vi "winHost.vi"() -> ()   [LabVIEW 2017]
uses:
  <vilib>/Utility/file.llb/Write Delimited Spreadsheet (DBL).vi
panel:
  in  "file path (dialog if empty)":path=path "C:/Users/adamg/Desktop/testdata137deg.csv"
  in  "Orientation":dbl
  in  "Force":dbl
  in  "Save":bool
  in  "stop":bool
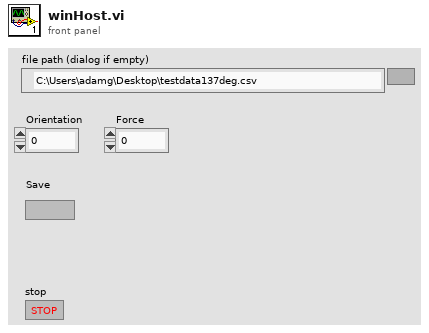
[diagram p1: front panel]
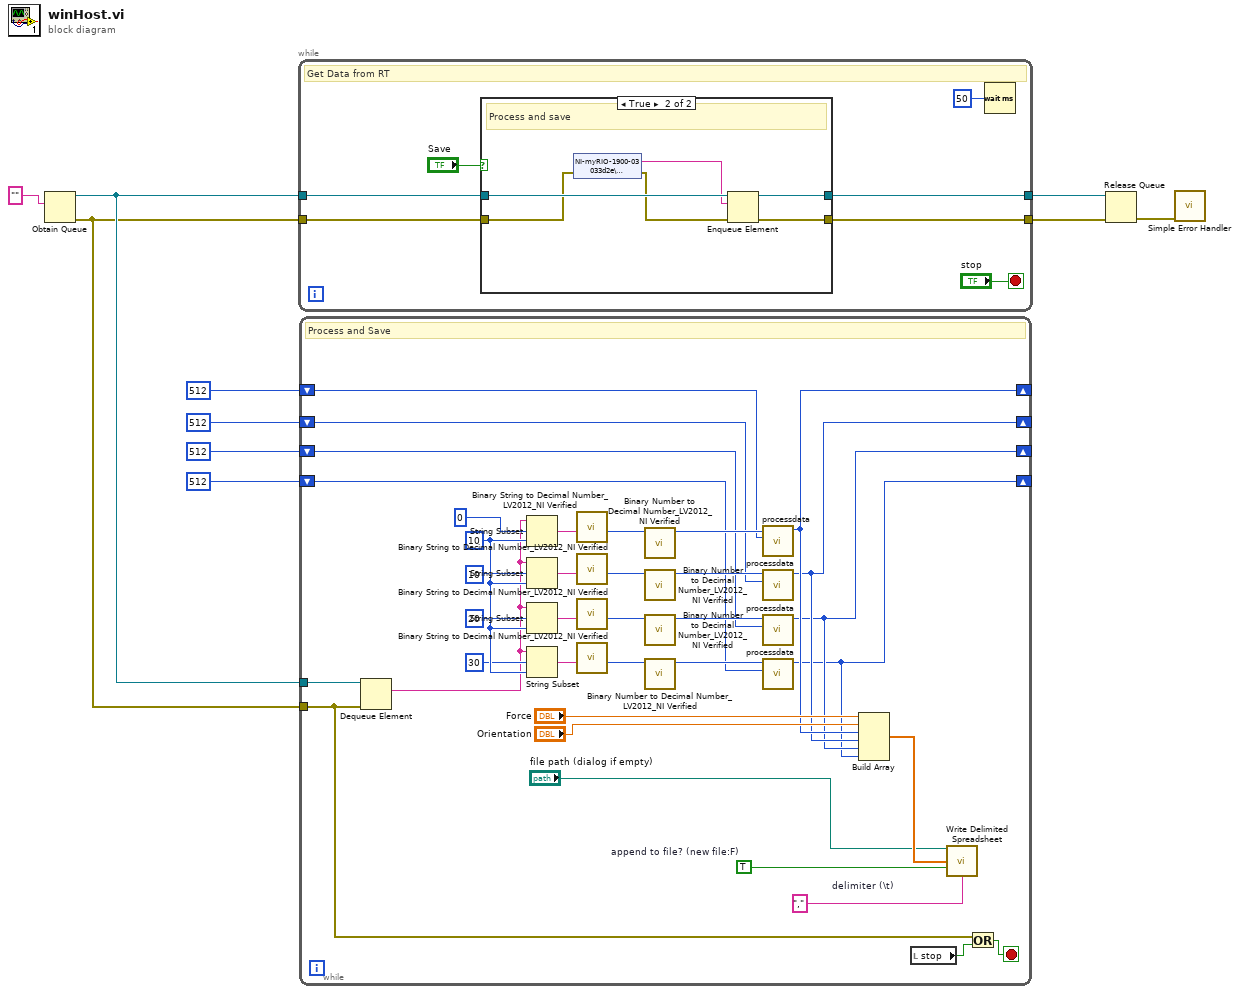
[diagram p0: block diagram]
diagram:
  n1 = Obtain Queue(element data type="") -> (queue out=w8:refnum<queue>, error out=w7:errorcluster)  [unwired: 4 in, 1 out]
  n2 = while {
    tunnel: w8 -> [w15]
    tunnel: w7 -> [w14]
    tunnel: [w13] -> w10
    tunnel: [w12] -> w9
    stop <- "stop" stop-if-true
    # "Get Data from RT"
    n3 = case shown="True" "Save" {
      tunnel: w15 -> [w19 w25]
      tunnel: w14 -> [w18 w22]
      tunnel: [w19 w21] -> w13
      tunnel: [w18 w20] -> w12
      frame False {
      }
      frame True {
        # "Process and save"
        n4 = shared-variable "NI-myRIO-1900-03033d2e\\sharedVariables.lvlib\\data"(error in=w22) -> (w24:string, error out=w23:errorcluster)
        n5 = Enqueue Element(queue=w25, element=w24, error in (no error)=w23) -> (queue out=w21:refnum<queue>, error out=w20:errorcluster)  [unwired: 1 in, 1 out]
      }
    }
    n6 = Wait (ms)(milliseconds to wait=u32 50) -> ()  [unwired: 1 out]
  }
  n7 = while {
    tunnel: w8 -> [w61]
    tunnel: w7 -> [w26]
    shift-right: [w32] -> _
    shift-left: 512 -> [w36]
    shift-right: [w31] -> _
    shift-left: 512 -> [w35]
    shift-right: [w30] -> _
    shift-left: 512 -> [w34]
    shift-right: [w29] -> _
    shift-left: 512 -> [w33]
    stop <- w27 stop-if-true
    w44 = ","  # delimiter (\t)
    w45 = TRUE  # append to file? (new file:F)
    w56 = 10 ("length (rest)")
    # "Process and Save"
    n8 = Dequeue Element(queue=w61, error in (no error)=w26) -> (element=w51:string)  [unwired: 1 in, 3 out]
    n9 = String Subset(string=w51, offset (0)=0, length (rest)=w56) -> (substring=w57:string)
    n10 = String Subset(string=w51, offset (0)=10 ("length (rest)"), length (rest)=w56) -> (substring=w58:string)
    n11 = String Subset(string=w51, offset (0)=20 ("length (rest)"), length (rest)=w56) -> (substring=w59:string)
    n12 = String Subset(string=w51, offset (0)=30 ("length (rest)"), length (rest)=w56) -> (substring=w60:string)
    n13 = call "Binary String to Decimal Number_LV2012_NI Verified.vi"("String"=w57) -> ("Number"=w50:u64)  [unwired: 10 in]
    n14 = call "Binary String to Decimal Number_LV2012_NI Verified.vi"("String"=w58) -> ("Number"=w49:u64)  [unwired: 10 in]
    n15 = call "Binary String to Decimal Number_LV2012_NI Verified.vi"("String"=w59) -> ("Number"=w48:u64)  [unwired: 10 in]
    n16 = call "Binary String to Decimal Number_LV2012_NI Verified.vi"("String"=w60) -> ("Number"=w47:u64)  [unwired: 10 in]
    n17 = call "Binary Number to Decimal Number_LV2012_NI Verified.vi"("Binary number"=w50) -> ("Decimal number"=w40:i32)  [unwired: 10 in]
    n18 = call "Binary Number to Decimal Number_LV2012_NI Verified.vi"("Binary number"=w49) -> ("Decimal number"=w39:i32)  [unwired: 10 in]
    n19 = call "Binary Number to Decimal Number_LV2012_NI Verified.vi"("Binary number"=w48) -> ("Decimal number"=w38:i32)  [unwired: 10 in]
    n20 = call "Binary Number to Decimal Number_LV2012_NI Verified.vi"("Binary number"=w47) -> ("Decimal number"=w37:i32)  [unwired: 10 in]
    n21 = call "processdata.vi"("oldrawin"=w36, "rawin"=w40) -> ("rawout2"=w32:i32)  [unwired: 9 in]
    n22 = call "processdata.vi"("oldrawin"=w35, "rawin"=w39) -> ("rawout2"=w31:i32)  [unwired: 9 in]
    n23 = call "processdata.vi"("oldrawin"=w34, "rawin"=w38) -> ("rawout2"=w30:i32)  [unwired: 9 in]
    n24 = call "processdata.vi"("oldrawin"=w33, "rawin"=w37) -> ("rawout2"=w29:i32)  [unwired: 9 in]
    n25 = Build Array("Force", "Orientation", w32, w31, w30, w29) -> (w46:dbl[])
    n26 = local read "stop"() -> (w28:bool)
    n27 = call-poly <vilib>:"Write Delimited Spreadsheet.vi"("file path (dialog if empty)"="file path (dialog if empty)", "1D data"=w46, "append to file? (new file:F)"=w45, "delimiter (\\t)"=w44) -> ()  [unwired: 10 in, 2 out]
    n28 = Or(x=w26, y=w28) -> (x .or. y?=w27:bool)
  }
  n29 = Release Queue(queue=w10, error in (no error)=w9) -> (error out=w5:errorcluster)  [unwired: 1 in, 2 out]
  n30 = call <vilib>:"Simple Error Handler.vi"("error in (no error)"=w5) -> ()  [unwired: 4 in, 5 out]
